vi "ZeroCAL_1.vi"(8 "error in":errorcluster, 11 "VISA in":refnum<visa-resource-name>) -> (0 "error out":errorcluster, 3 "VISA out":refnum<visa-resource-name>)   [LabVIEW 2020, in "Keysight.lvlib"]
uses:
  Keysight.lvlib
panel:
  out "Response":string
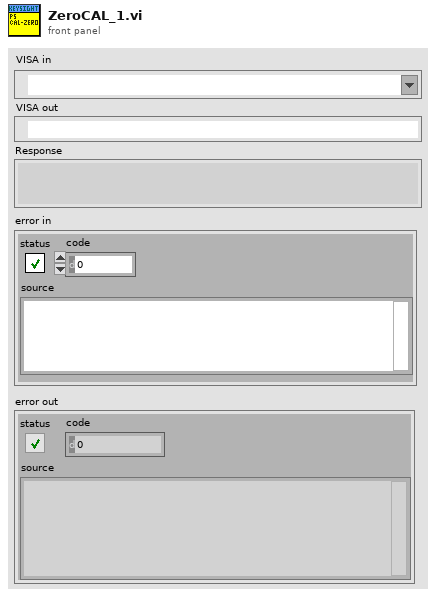
[diagram p1: front panel]
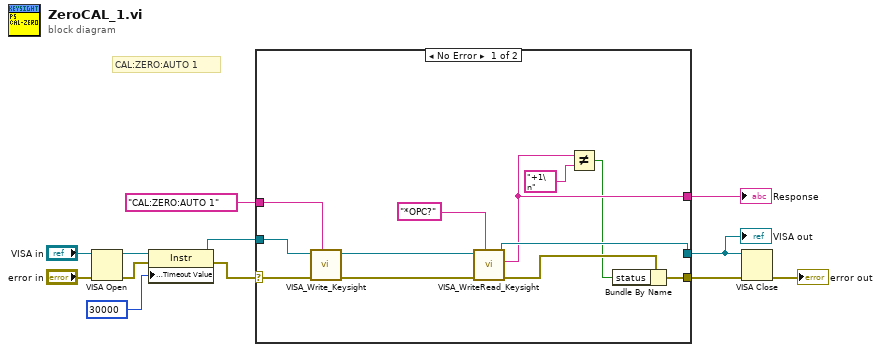
[diagram p0: block diagram]
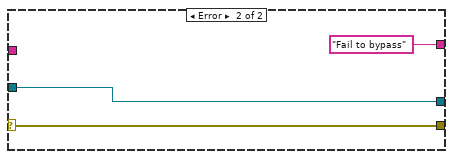
[diagram p2: hidden frame]
diagram:
  # "CAL:ZERO:AUTO 1"
  n1 = VISA Open(error in (no error)="error in", VISA resource name="VISA in") -> (VISA resource name=w5:refnum<visa-resource-name>, error out=w7:errorcluster)  [unwired: 3 in]
  n2 = property on="Property Node" class="Instr"(reference=w5, error in=w7, "General Settings:Timeout Value"=u32 30000) -> (reference out=w9:refnum<visa-resource-name>, error out=w10:errorcluster)
  n3 = case shown="No Error" w10 {
    selector: w10 -> [w22 w27]
    tunnel: [w14 w27] -> w4
    tunnel: [w19 w26] -> w2
    tunnel: "CAL:ZERO:AUTO 1" ("write buffer") -> [w24 _]
    tunnel: w9 -> [w23 w26]
    tunnel: [w17 "Fail to bypass" ("Response")] -> w1
    frame No Error {
      n4 = call "VISA_Write_Keysight.vi"("VISA CMD"=w24, "error in"=w22, "VISA in"=w23) -> ("error out"=w21:errorcluster, "VISA out"=w20:refnum<visa-resource-name>)  [unwired: 7 in]
      n5 = call "VISA_WriteRead_Keysight.vi"("VISA_CMD"="*OPC?" ("write buffer"), "error in"=w21, "VISA in"=w20) -> ("error out"=w16:errorcluster, "Response"=w17:string, "VISA out"=w19:refnum<visa-resource-name>)  [unwired: 6 in]
      n6 = Not Equal?(x=w17, y="+1\n" ("Response 2")) -> (x != y?=w15:bool)
      n7 = Bundle By Name(cluster=w16, "status"=w15) -> (w14:errorcluster)
    }
    frame Error {
    }
  }
  "VISA out" <- w2
  "Response" <- w1
  n8 = VISA Close(VISA resource name=w2, error in (no error)=w4) -> (error out=→"error out":errorcluster)
